vi "AT Get Int A.vi"(8 "error in (no error)":errorcluster, 10 "Feature":string, 11 "Handle":i32) -> (0 "error out":errorcluster, 2 "Value":i64, 3 "Status":i32)   [LabVIEW 2019]
doc: "Get Int\n\nOutput:\n I32 Status\n\nInput:\n I32 Handle\n String Feature\n I64 Value\n\nThe function will return the current value for the specified feature. The function will return an error if the feature is currently not readable or if the specified feature is either not an integer feature or is not implemented by the camera."
uses:
  atcoreA.dll
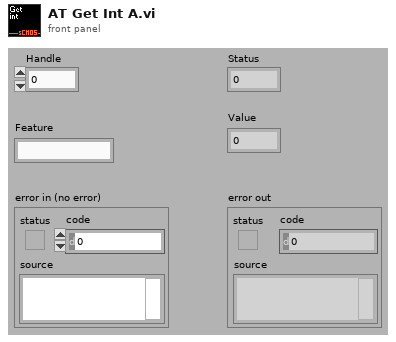
[diagram p1: front panel]
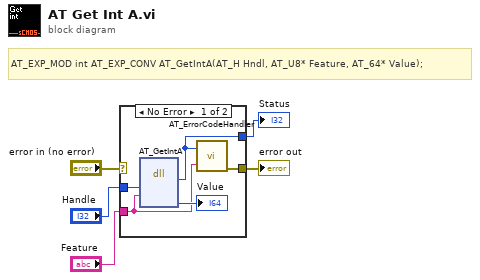
[diagram p0: block diagram]
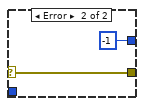
[diagram p2: hidden frame]
diagram:
  # "AT_EXP_MOD int AT_EXP_CONV AT_GetIntA(AT_H Hndl, AT_U8* Feature, AT_64* Value);"
  n1 = case shown="No Error" "error in (no error)" {
    selector: "error in (no error)" -> [_ w12]
    tunnel: [w7 -1] -> w5
    tunnel: "Handle" -> [w10 _]
    tunnel: "Feature" -> [w6 _]
    tunnel: [w8 w12] -> w1
    frame No Error {
      n2 = dll-call lib="atcoreA.dll" fn="AT_GetIntA"("Handle"=w10, "Feature"=w6) -> ("Status"=w7:i32, "Value"=→"Value":i64)  [unwired: 6 in, 2 out]
      n3 = call "AT_ErrorCodeHandler.vi"("Error"=w7, "Feature Name"=w6) -> ("error out"=w8:errorcluster)  [unwired: 5 in]
    }
    frame Error {
    }
  }
  "Status" <- w5
  "error out" <- w1
